vi "Create.vi"(10 "Events":T1[](array[typedef])) -> (3 "EventsValue out":refnum<class "EventsValue.lvclass">)   [LabVIEW 2020, in "Volatus.lvlib" / "EventsValue.lvclass"]
uses:
  EventsValue.lvclass
  EventsValue.lvclass/EventsValue.ctl
  Event Level.ctl
  Volatus.lvlib
  Event.ctl
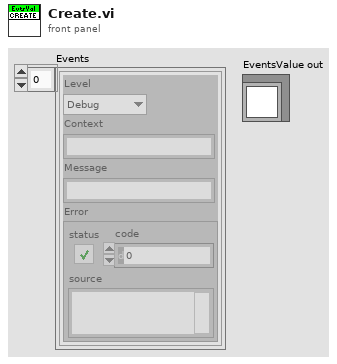
[diagram p1: front panel]
types:
  T1 = typedef "Volatus.lvlib/Event.ctl" = cluster{"Level":T2, "Context":string, "Message":string, "Error":errorcluster}
  T2 = typedef "Volatus.lvlib/Event Level.ctl" = enum16{"Debug", "Info", "Warning", "Error"}
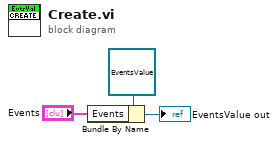
[diagram p0: block diagram]
diagram:
  n1 = Bundle By Name(cluster=refnum<class "EventsValue.lvclass"> refnum ("EventsValue in"), "Events"="Events") -> (→"EventsValue out":refnum<class "EventsValue.lvclass">)
